vi "IsNull.vi"(4 "ProductA":refnum<class "ProductA.lvclass">) -> (1 "isNull":bool)   [LabVIEW 2020, in "FactoryMethod.lvlib" / "FactoryMethodLazyEvaluation.lvlib" / "ProductA.lvclass"]
uses:
  ProductA.lvclass
  ProductA.lvclass/ProductA.ctl
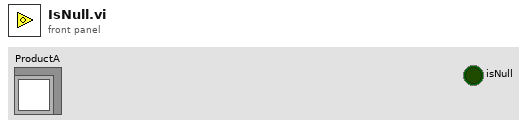
[diagram p1: front panel]
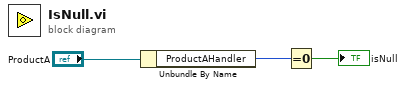
[diagram p0: block diagram]
diagram:
  n1 = Unbundle By Name("ProductA") -> ("ProductAHandler"=w1:u32)
  n2 = Equal To 0?(x=w1) -> (x = 0?=→"isNull":bool)
